vi "Example Callback - Current Callback.vi"(4 "Current":refnum<user-event>, 5 "Event Data":cluster{"sender":refnum<k24>, "current":i16}, 6 "Control Ref":refnum<k24>, 7 "Event Common Data":T1) -> ()   [LabVIEW 2013]
uses:
  C:/tf/play/labview/Tinkerforge.dll
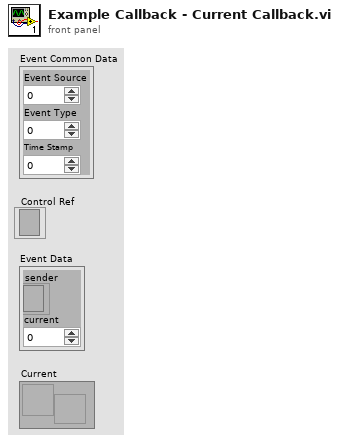
[diagram p1: front panel]
types:
  T1 = cluster{"Event Source":i32, "Event Type":u32, "Time Stamp":u32}
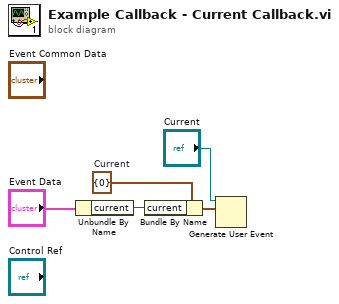
[diagram p0: block diagram]
diagram:
  w3 = cluster{"current":i16} {"current"=0}  # Current
  n1 = Unbundle By Name("Event Data") -> ("current"=w4:i16)
  n2 = Bundle By Name(cluster=w3, "current"=w4) -> (w2:cluster{"current":i16})
  n3 = Generate User Event(user event="Current", event data cluster=w2) -> ()  [unwired: 2 in, 2 out]
